vi "is_ds_open.vi"(9 "error in (no error)":errorcluster) -> (1 "error out":errorcluster, 2 "ds open?":bool)   [LabVIEW 2015]
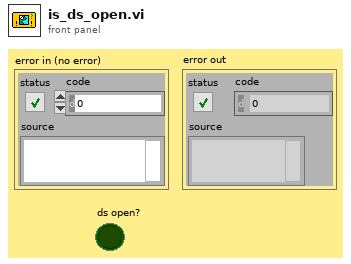
[diagram p1: front panel]
types:
  T1 = enum16{"Read", "Write", "ReadWrite", "BufferedRead", "BufferedReadWrite"}
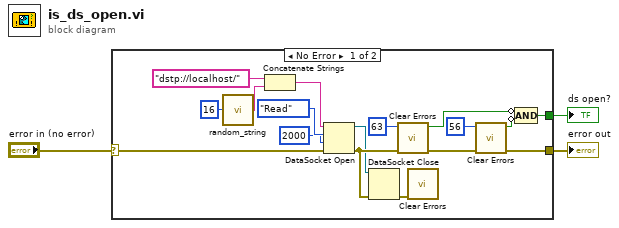
[diagram p0: block diagram]
diagram:
  n1 = case shown="No Error" "error in (no error)" {
    selector: "error in (no error)" -> [w13 w21]
    tunnel: [w4 w21] -> w3
    tunnel: [w8 _] -> w1
    frame No Error {
      n2 = call "random_string.vi"("length"=16) -> ("random string"=w18:string)  [unwired: 8 in]
      n3 = Concatenate Strings("dstp://localhost/" ("URL"), w18) -> (w16:string)
      n4 = DataSocket Open(8:w13, 9:2000 ("ms timeout (10000)"), 10:T1."Read" ("mode"), 11:w16) -> (0:w7:errorcluster, 3:w6:refnum<k13>)
      n5 = DataSocket Close(8:w7, 11:w6) -> (0:w5:errorcluster)  [unwired: 1 in, 1 out]
      n6 = call <vilib>:"Clear Errors.vi"("error in (no error)"=w7, "specific error code to clear (0: all)"=63) -> ("error out"=w12:errorcluster, "specific error cleared?"=w10:bool)  [unwired: 4 in]
      n7 = call <vilib>:"Clear Errors.vi"("error in (no error)"=w5) -> ()  [unwired: 5 in, 2 out]
      n8 = call <vilib>:"Clear Errors.vi"("error in (no error)"=w12, "specific error code to clear (0: all)"=56) -> ("error out"=w4:errorcluster, "specific error cleared?"=w9:bool)  [unwired: 4 in]
      n9 = Compound Arithmetic op=AND(invert w10, invert w9) -> (w8:bool)
    }
    frame Error {
    }
  }
  "error out" <- w3
  "ds open?" <- w1
